vi "Check coord input.vi"(10 "coordIn":string, 11 "RA=T, default: F=DEC":bool) -> (2 "coordOut":string, 3 "valid":bool)   [LabVIEW 2018]
uses:
  <vilib>/regexp/Match Regular Expression.xnode
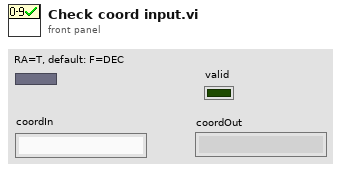
[diagram p1: front panel]
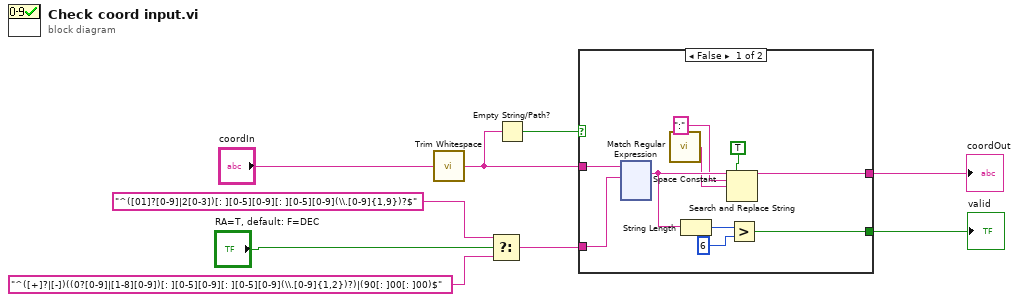
[diagram p0: block diagram]
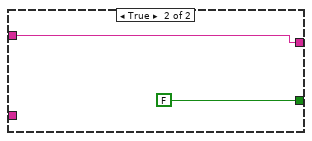
[diagram p2: hidden frame]
diagram:
  n1 = call <vilib>:"Trim Whitespace.vi"("string"="coordIn") -> ("trimmed string"=w8:string)  [unwired: 1 in]
  n2 = Select(t="^([01]?[0-9]|2[0-3])[: ][0-5][0-9][: ][0-5][0-9](\\.[0-9]{1,9})?$" ("Regular Expression"), s="RA=T, default: F=DEC", f="^([+]?|[-])((0?[0-9]|[1-8][0-9])[: ][0-5][0-9][: ][0-5][0-9](\\.[0-9]{1,2})?)|(90[: ]00[: ]00)$" ("Regular Expression")) -> (s? t:f=w2:string)
  n3 = Empty String/Path?(string/path=w8) -> (empty?=w7:bool)
  n4 = case shown="False" w7 {
    tunnel: w8 -> [w18 w134]
    tunnel: w2 -> [w19 _]
    tunnel: [w17 FALSE] -> w6
    tunnel: [w10 w134] -> w1
    frame False {
      n5 = xnode "Match Regular Expression"("input string"=w18, "regular expression"=w19) -> ("whole match"=w14:string)  [unwired: 4 in, 4 out]
      n6 = call <vilib>:"Space Constant.vi"() -> ("String"=w12:string)
      n7 = String Length(string=w14) -> (length=w16:i32)
      n8 = Search and Replace String(replace all?=TRUE ("replace all? (F)"), input string=w14, search string=":", replace string=w12) -> (result string=w10:string)  [unwired: 4 in, 3 out]
      n9 = Greater?(x=w16, y=6) -> (0:w17:bool)
    }
    frame True {
    }
  }
  "valid" <- w6
  "coordOut" <- w1
